vi "KE622x -- 2182 -A Reset.vi"(0 "622x Resource In":refnum<visa-resource-name>, 1 "Check For SCPI Errors? (T)":bool=TRUE, 11 "error in (no error)":errorcluster) -> (4 "622x Resource Out (dupl)":refnum<visa-resource-name>, 15 "error out":errorcluster)   [LabVIEW 2019, in "Keithley 622x.lvlib"]
doc: "Performs a reset of the 2182/2182A connected to the 622x over the RS232 link."
uses:
  Keithley 622x.lvlib
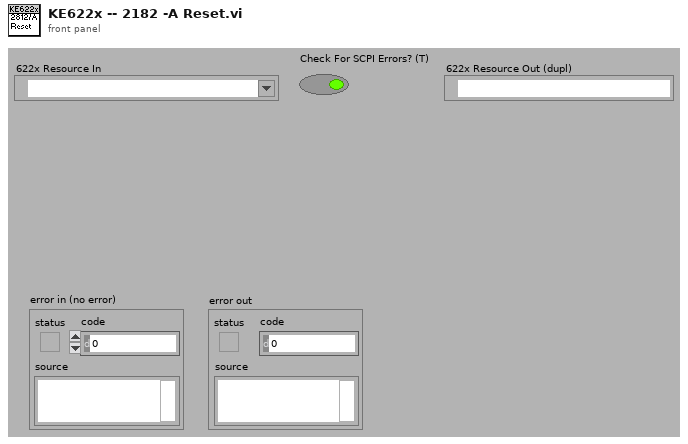
[diagram p1: front panel]
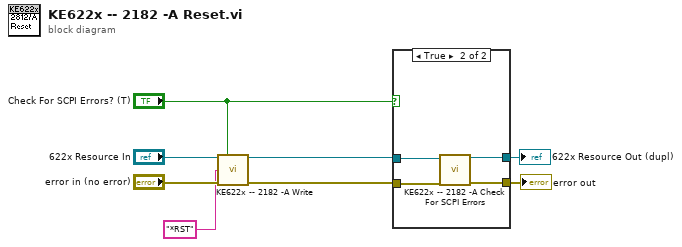
[diagram p0: block diagram]
diagram:
  n1 = call "KE622x -- 2182 -A Write.vi"("Resource In"="622x Resource In", "Check For SCPI Errors? (T)"="Check For SCPI Errors? (T)", "2182-A Write String"="*RST", "error in (no error)"="error in (no error)") -> ("Resource Out (dupl)"=w6:refnum<visa-resource-name>, "error out"=w2:errorcluster)  [unwired: 10 in]
  n2 = case shown="True" "Check For SCPI Errors? (T)" {
    tunnel: w6 -> [w10 w14]
    tunnel: w2 -> [w9 w13]
    tunnel: [w10 w12] -> w4
    tunnel: [w9 w11] -> w3
    frame False {
    }
    frame True {
      n3 = call "KE622x -- 2182 -A Check For SCPI Errors.vi"("VISA Resource In"=w14, "error in (no error)"=w13) -> ("VISA Resource Out (dupl)"=w12:refnum<visa-resource-name>, "error out"=w11:errorcluster)  [unwired: 10 in, 2 out]
    }
  }
  "622x Resource Out (dupl)" <- w4
  "error out" <- w3
